vi "create.from_array.vi"(10 "labels":string[](array[string])) -> (3 "labels out":refnum<class "labels.lvclass">)   [LabVIEW 2020, in "nominal types.lvlib" / "labels.lvclass"]
uses:
  labels.lvclass
  labels.lvclass/labels.ctl
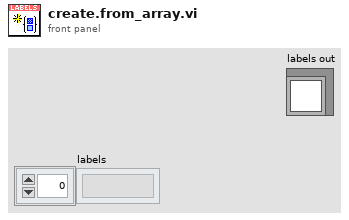
[diagram p1: front panel]
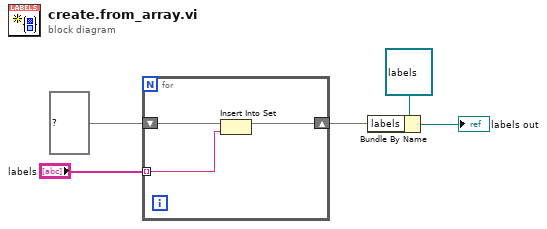
[diagram p0: block diagram]
diagram:
  n1 = for {
    shift-right: [w7] -> w3
    shift-left: set{string} {} ("labels") -> [w8]
    tunnel: "labels" -> [w6] mode=indexing
    n2 = Insert Into Set(10:w6, 11:w8) -> (3:w7:set{string})  [unwired: 1 out]
  }
  n3 = Bundle By Name(cluster=refnum<class "labels.lvclass"> refnum ("properties out"), "labels"=w3) -> (→"labels out":refnum<class "labels.lvclass">)
